vi "Specific Line Output.vi"(5 "turn over address":u8=64, 6 "chip select":enum16{"1st chip", "2nd chip"}(ring), 7 "end address":u8, 8 "error in (no error)":errorcluster, 9 "start address":u8, 10 "character codes":u8[](array[numeric]), 11 "cluster of private data in":T1={"FPGA VI Reference"=refnum, "device index"=0, "screen size"=enum."8x1", "font size"=enum."5x8", "auto wrap"=FALSE, "alignment"=enum."None", "number of line"=enum."2 lines", "shift 0"=0, "entry mode 0"=enum."increment & no shift", "shift 1"=0, "entry mode 1"=enum."increment & no shift"}) -> (0 "error out":errorcluster, 3 "cluster of private data out":T1={"FPGA VI Reference"=refnum, "device index"=0, "screen size"=enum."8x1", "font size"=enum."5x8", "auto wrap"=FALSE, "alignment"=enum."None", "number of line"=enum."2 lines", "shift 0"=0, "entry mode 0"=enum."increment & no shift", "shift 1"=0, "entry mode 1"=enum."increment & no shift"})   [LabVIEW 2017, in "HD44780.lvclass"]
uses:
  HD44780.lvclass
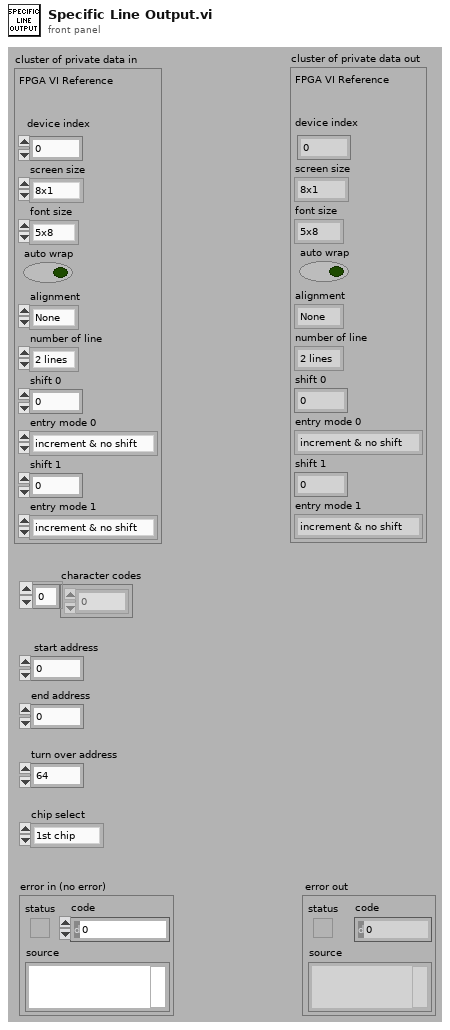
[diagram p1: front panel]
types:
  T1 = cluster{"FPGA VI Reference":refnum<k20>, "device index":i8, "screen size":enum8{"8x1", "8x2", "12x4", "16x1", "16x2", "16x4", "20x1", "20x2", "20x4", "24x1", "24x2", "40x2", "40x4"}, "font size":enum8{"5x8", "5x10"}, "auto wrap":bool, "alignment":enum16{"None", "Left", "Center", "Right"}, "number of line":enum8{"1 line", "2 lines"}, "shift 0":i8, "entry mode 0":enum8{"increment & no shift", "increment & shift", "decrement & no shift", "decrement & shift"}, "shift 1":i8, "entry mode 1":enum8{"increment & no shift", "increment & shift", "decrement & no shift", "decrement & shift"}}
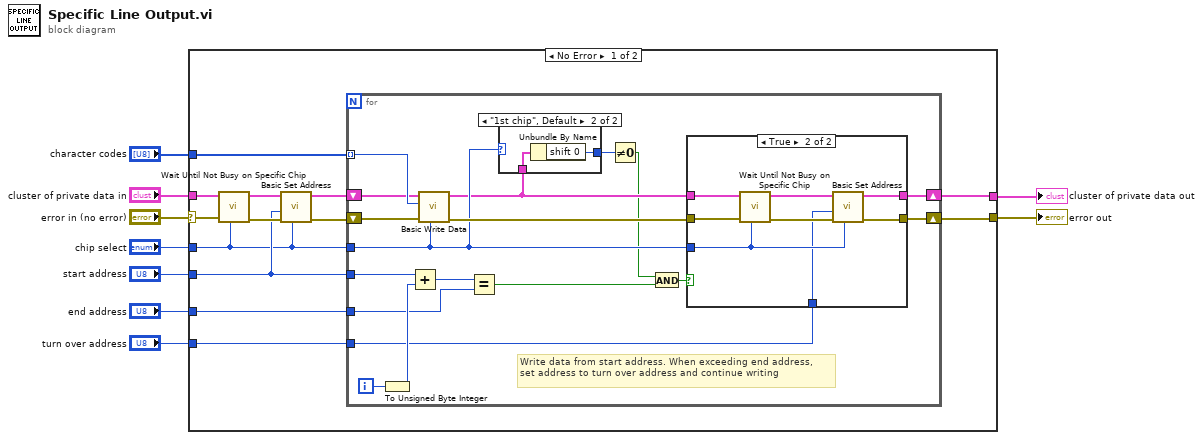
[diagram p0: block diagram]
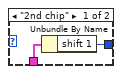
[diagram p2: hidden frame]
diagram:
  n1 = case shown="No Error" "error in (no error)" {
    selector: "error in (no error)" -> [w16 w56]
    tunnel: "chip select" -> [w10 _]
    tunnel: [w19 w55] -> w7
    tunnel: "cluster of private data in" -> [w17 w55]
    tunnel: [w18 w56] -> w1
    tunnel: "turn over address" -> [w20 _]
    tunnel: "character codes" -> [w22 _]
    tunnel: "start address" -> [w11 _]
    tunnel: "end address" -> [w21 _]
    frame No Error {
      n2 = call "Wait Until Not Busy on Specific Chip.vi"("chip select  (1st chip)"=w10, "error in (no error)"=w16, "cluster of private data in"=w17) -> ("error out"=w14:errorcluster, "cluster of private data out"=w15:T1)  [unwired: 7 in]
      n3 = call "Basic Set Address.vi"("chip select  (1st chip)"=w10, "error in (no error)"=w14, "address (0, 0)"=w11, "cluster of private data in"=w15) -> ("error out"=w12:errorcluster, "cluster of private data out"=w13:T1)  [unwired: 6 in]
      n4 = for {
        shift-right: [w30] -> w18
        shift-left: w12 -> [w35]
        shift-right: [w31] -> w19
        shift-left: w13 -> [w33]
        tunnel: w22 -> [w34] mode=indexing
        tunnel: w10 -> [w28]
        tunnel: w11 -> [w39]
        tunnel: w21 -> [w37]
        tunnel: w20 -> [w29]
        i -> [w40]
        # "Write data from start address. When exceeding end address,\nset address to turn over address and continue writing"
        n5 = To Unsigned Byte Integer(number=w40) -> (unsigned 8bit integer=w38:u8)
        n6 = Add(x=w39, y=w38) -> (x+y=w36:u8)
        n7 = call "Basic Write Data.vi"("chip select  (1st chip)"=w28, "error in (no error)"=w35, "character code"=w34, "cluster of private data in"=w33) -> ("error out"=w32:errorcluster, "cluster of private data out"=w27:T1)  [unwired: 6 in]
        n8 = Equal?(x=w36, y=w37) -> (x = y?=w24:bool)
        n9 = case shown="\"1st chip\", Default" w28 {
          tunnel: w27 -> [w42 w44]
          tunnel: [w41 w43] -> w26
          frame "2nd chip" {
            n10 = Unbundle By Name(w42) -> ("shift 1"=w41:i8)
          }
          frame "1st chip", Default {
            n11 = Unbundle By Name(w44) -> ("shift 0"=w43:i8)
          }
        }
        n12 = Not Equal To 0?(x=w26) -> (x != 0?=w23:bool)
        n13 = And(x=w23, y=w24) -> (x .and. y?=w25:bool)
        n14 = case shown="True" w25 {
          tunnel: w27 -> [w46 w54]
          tunnel: w32 -> [w45 w53]
          tunnel: [w46 w50] -> w31
          tunnel: [w45 w49] -> w30
          tunnel: w28 -> [_ w48]
          tunnel: w29 -> [_ w47]
          frame False {
          }
          frame True {
            n15 = call "Wait Until Not Busy on Specific Chip.vi"("chip select  (1st chip)"=w48, "error in (no error)"=w53, "cluster of private data in"=w54) -> ("error out"=w51:errorcluster, "cluster of private data out"=w52:T1)  [unwired: 7 in]
            n16 = call "Basic Set Address.vi"("chip select  (1st chip)"=w48, "error in (no error)"=w51, "address (0, 0)"=w47, "cluster of private data in"=w52) -> ("error out"=w49:errorcluster, "cluster of private data out"=w50:T1)  [unwired: 6 in]
          }
        }
      }
    }
    frame Error {
    }
  }
  "cluster of private data out" <- w7
  "error out" <- w1
